vi "Shutdown.vi"(8 "error in (no error)":errorcluster, 11 "DigitalIO in":refnum<class "DigitalIO.lvclass">) -> (0 "error out":errorcluster, 3 "DigitalIO out":refnum<class "DigitalIO.lvclass">)   [LabVIEW 2018, in "DigitalIO.lvlib" / "DigitalIO.lvclass"]
uses:
  DigitalIO.lvclass
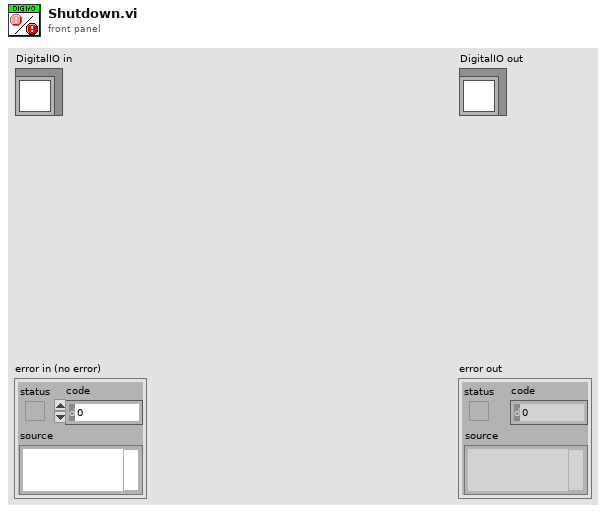
[diagram p1: front panel]
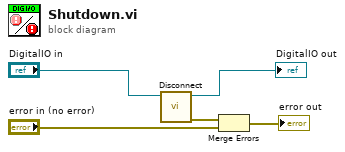
[diagram p0: block diagram]
diagram:
  n1 = call-dynamic "Disconnect.vi"("DigitalIO in"="DigitalIO in") -> ("error out"=w4:errorcluster, "DigitalIO out"=→"DigitalIO out":refnum<class "DigitalIO.lvclass">)  [unwired: 9 in]
  n2 = Merge Errors(w4, "error in (no error)") -> (→"error out":errorcluster)
